vi "Delete Float64 DVR.vi"(8 "error in (no error)":errorcluster, 11 "Float64 DVR in":refnum<data-value>) -> (0 "error out":errorcluster, 3 "Float64 out":refnum<class "Float64.lvclass">)   [LabVIEW 2015, in "MDSplus.lvlib" / "Float64.lvclass"]
uses:
  <vilib>/MDSplus/Classes/Data_Class/Scalar_Class/Float64_Class/Float64.lvclass
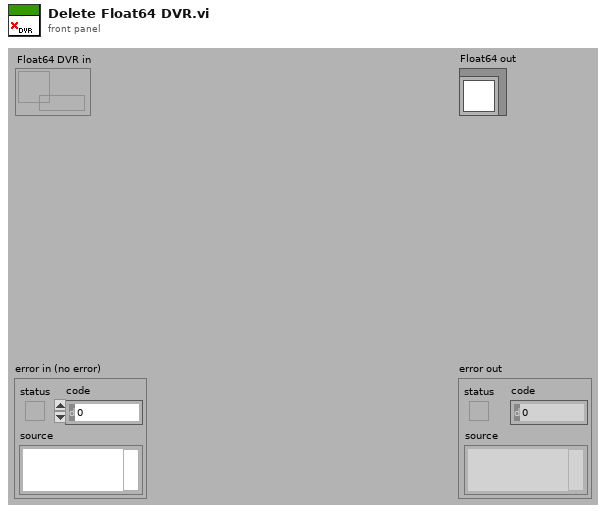
[diagram p1: front panel]
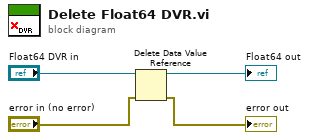
[diagram p0: block diagram]
diagram:
  n1 = Delete Data Value Reference(data value reference="Float64 DVR in", error in="error in (no error)") -> (data value=→"Float64 out":refnum<class "Float64.lvclass">, error out=→"error out":errorcluster)
